vi "CONV 1D Fractional Array to String.vi"(0 "1-D Fractional":dbl[](array[numeric]) format="%.2f", 1 "Delimiter (,)":string=",", 5 "Precision (2)":i32=2) -> (6 "String":string)   [LabVIEW 2012]
doc: "This routine converts a 1-D DBL Precision Fractional Array into a string list. The delimiter may be one or more characters."
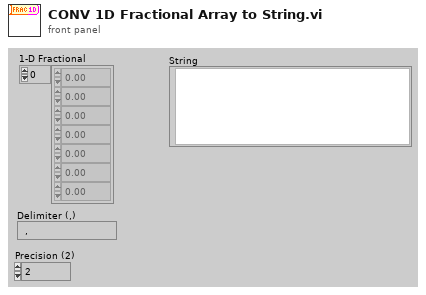
[diagram p1: front panel]
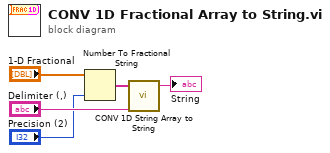
[diagram p0: block diagram]
diagram:
  n1 = Number To Fractional String(number="1-D Fractional", precision (6)="Precision (2)") -> (F-format string=w4:string[])  [unwired: 2 out]
  n2 = call "CONV 1D String Array to String.vi"("1-D String"=w4, "Delimiter (,)"="Delimiter (,)") -> ("String"=→"String":string)  [unwired: 7 out]
